vi "Handle dotNet Execptions.vi"(8 "error in (no error)":errorcluster, 11 ".NET Refnum in":refnum<k24>) -> (0 "error out":errorcluster)   [LabVIEW 2020, in "WebView.lvclass"]
uses:
  WebView.lvclass
  DotNet Execption Message--cluster.ctl
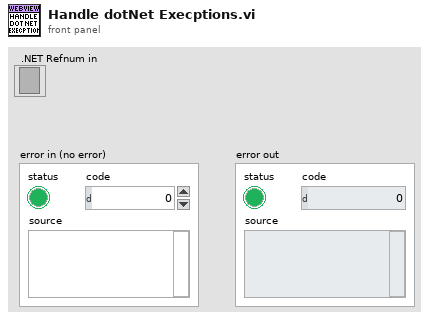
[diagram p1: front panel]
types:
  T1 = typedef "WebView.lvclass/DotNet Execption Message--cluster.ctl" = cluster{"Message":string, "Source":string, "StackTrace":string}
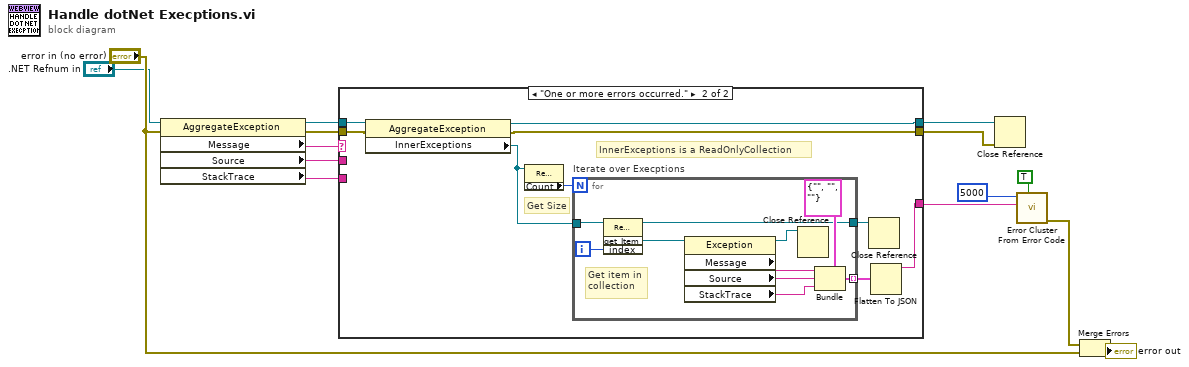
[diagram p0: block diagram]
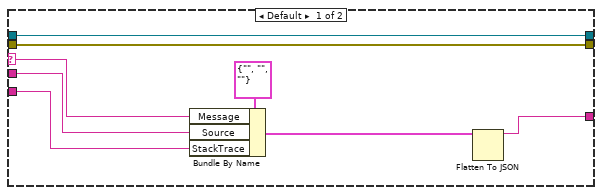
[diagram p2: hidden frame]
diagram:
  n1 = property class="AggregateException"(reference=".NET Refnum in", error in="error in (no error)") -> (reference out=w13:refnum<k24>, error out=w11:errorcluster, "Message"=w7:string, "Source"=w9:string, "StackTrace"=w8:string)
  n2 = case shown="\"One or more errors occurred.\"" w7 {
    selector: w7 -> [w21 _]
    tunnel: w8 -> [w19 _]
    tunnel: w9 -> [w20 _]
    tunnel: [w18 w24] -> w4
    tunnel: [w16 w27] -> w10
    tunnel: w11 -> [w16 w29]
    tunnel: [w15 w28] -> w12
    tunnel: w13 -> [w15 w30]
    frame Default {
      n3 = Bundle By Name(cluster=T1 {"Message"="", "Source"="", "StackTrace"=""}, "Message"=w21, "Source"=w20, "StackTrace"=w19) -> (w17:T1)
      n4 = Flatten To JSON(anything=w17) -> (JSON string=w18:string)  [unwired: 2 in, 1 out]
    }
    frame "One or more errors occurred." {
      # "Get Size"
      # "InnerExceptions is a ReadOnlyCollection"
      n5 = property class="AggregateException"(reference=w30, error in=w29) -> (reference out=w28:refnum<k24>, error out=w27:errorcluster, "InnerExceptions"=w26:refnum<k24>)
      n6 = property class="ReadOnlyCollection`1[[System.Ex"(reference=w26) -> ("Count"=w31:i32)  [unwired: 1 in, 2 out]
      n7 = for "Iterate over Execptions" {
        N: w31 -> [_]
        tunnel: w26 -> [w41]
        tunnel: [w34] -> w25 mode=indexing
        tunnel: [w33] -> w23
        i -> [w39]
        # "Get item in\ncollection"
        n8 = invoke class="ReadOnlyCollection`1[[System.Ex" method="get_Item"(reference=w41, "index"=w39) -> (reference out=w33:refnum<k24>, "get_Item"=w40:refnum<k24>)  [unwired: 2 in, 2 out]
        n9 = property class="Exception"(reference=w40) -> (reference out=w32:refnum<k24>, "Message"=w37:string, "Source"=w36:string, "StackTrace"=w35:string)  [unwired: 1 in, 1 out]
        n10 = Close Reference(reference=w32) -> ()  [unwired: 1 in, 1 out]
        n11 = Bundle(cluster=T1 {"Message"="", "Source"="", "StackTrace"=""}, "Message"=w37, "Source"=w36, "StackTrace"=w35) -> (w34:T1)
      }
      n12 = Close Reference(reference=w23) -> ()  [unwired: 1 in, 1 out]
      n13 = Flatten To JSON(anything=w25) -> (JSON string=w24:string)  [unwired: 2 in, 1 out]
    }
  }
  n14 = Close Reference(reference=w12, error in (no error)=w10) -> ()  [unwired: 1 out]
  n15 = call <vilib>:"Error Cluster From Error Code.vi"("show call chain? (False)"=TRUE, "error message (\"\")"=w4, "error code (0)"=5000 ("code")) -> ("error out"=w1:errorcluster)  [unwired: 6 in]
  n16 = Merge Errors(w1, "error in (no error)") -> (→"error out":errorcluster)
